vi "Smoothing.vi"(9 "Data in":T1) -> (1 "Data out":T1)   [LabVIEW 2013]
uses:
  xcontrol/Interface VIs/Interface typedefs/Interface-Data array.ctl
  xcontrol/Interface VIs/Interface typedefs/Interface-Data format definition.ctl
  xcontrol/Typedefs/Xctl-XY data type definition.ctl
  xcontrol/Typedefs/Xctrl-ROI type enum.ctl
  <vilib>/Analysis/3filter.llb/IIR Filter with I.C. (DBL).vi
  Global variables/gl_Functional Imaging-Global variables.vi
  <vilib>/Analysis/NI_AALBase.lvlib
  xcontrol/XGrapher.xctl
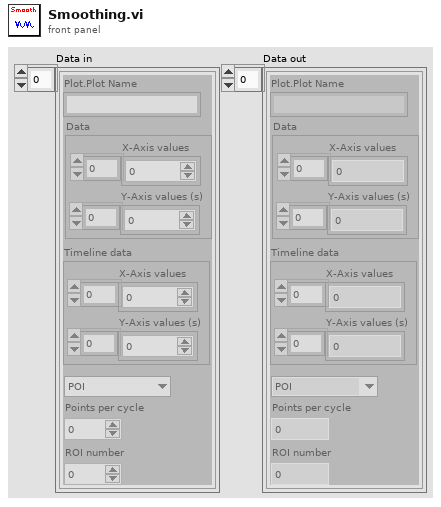
[diagram p1: front panel]
types:
  T1 = typedef "Interface-Data array.ctl" = T2[]
  T2 = typedef "Interface-Data format definition.ctl" = cluster{"Plot.Plot Name":string, "Data":T3, "Timeline data":T3, "Type":T4, "Points per cycle":u16, "ROI number":u16}
  T3 = typedef "XGrapher.xctl/Xctl-XY data type definition.ctl" = cluster{"X-Axis values":sgl[], "Y-Axis values (s)":i32[]}
  T4 = typedef "Xctrl-ROI type enum.ctl" = enum16{"POI", "Mini-scan", "Group"}
  T5 = typedef "Functional Imging UI Refs.ctl" = cluster{"Menu ref":refnum<k9>, "Image control":refnum<vi>, "VI ref":refnum<vi>, "XGrapher":refnum<vi>, "Smoothing":refnum<vi>, "POI Averaging":refnum<vi>, "Normalize":refnum<vi>, "POI data points in each trial":refnum<vi>, "Channel":refnum<vi>, "Experiment data folder path":refnum<vi>, "[ROI vis]":refnum<vi>, "[Groups] visbl":T6, "Group Name":refnum<vi>, "POI index":refnum<vi>, "Trial No.":refnum<vi>, "Intensity Zoom":refnum<vi>, "Trial Cursor Enabled":refnum<vi>, "Number of Trials (ind 1)":refnum<vi>, "Number of Trials (ind 2)":refnum<vi>, "MiniScans Available":refnum<vi>, "POI Available":refnum<vi>, "Defer graph updates":refnum<vi>, "Waveform selector":refnum<vi>, "#of selected POI":refnum<vi>, "#of selected MiniScans":refnum<vi>, "#of selected groups":refnum<vi>, "Max Z-Projection":refnum<vi>, "Z-Plane Selector":refnum<vi>, "Index of miniscan point to visualise":refnum<vi>, "ROI vis. mode":refnum<vi>, "Total # of points":refnum<vi>, "Index of group clicked on":refnum<vi>, "Pane 1":refnum<vi>, "Pane 2":refnum<vi>, "Pane 3":refnum<vi>, "Pane 4":refnum<vi>, "Pane 5":refnum<vi>, "Pane 6":refnum<vi>, "Deselect all ROI":refnum<vi>, "Deselect all groups":refnum<vi>}
  T6 = typedef "Groups array referecne.ctl" = refnum<vi>
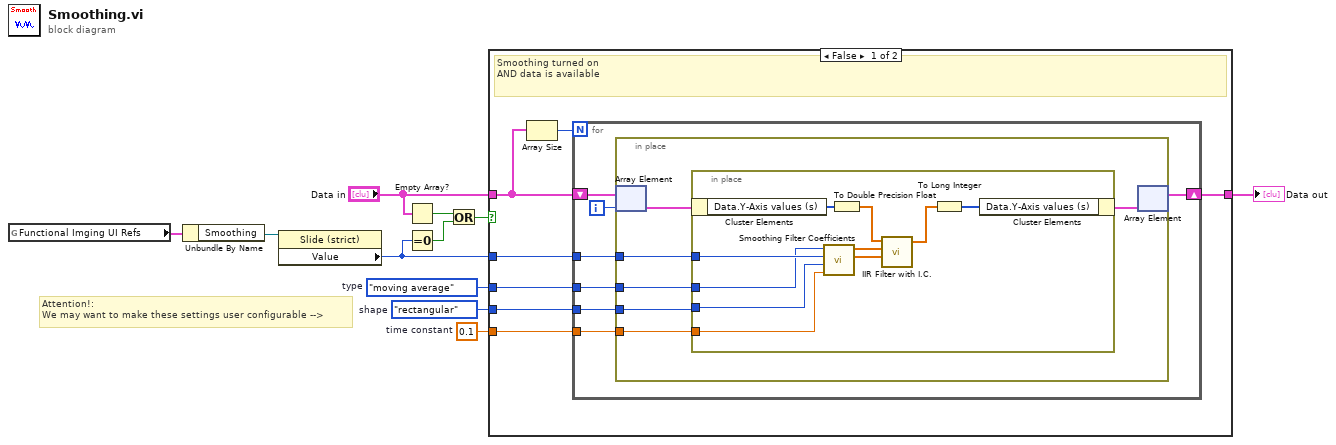
[diagram p0: block diagram]
diagram:
  w2 = 0.1  # time constant
  w3 = enum16{"rectangular", "triangular"}."rectangular"  # shape
  w4 = enum16{"moving average", "exponential"}."moving average"  # type
  # "Attention!:\nWe may want to make these settings user configurable -->"
  n1 = global read "gl_Functional Imaging-Global variables.vi" "Functional Imging UI Refs"() -> (w1:T5)
  n2 = Unbundle By Name(w1) -> ("Smoothing"=w11:refnum<vi>)
  n3 = property on="Property Node" class="Slide (strict)"(reference=w11) -> ("Value"=w5:i32)  [unwired: 1 in, 2 out]
  n4 = Empty Array?(array="Data in") -> (empty?=w8:bool)
  n5 = Equal To 0?(x=w5) -> (x = 0?=w9:bool)
  n6 = Or(x=w8, y=w9) -> (x .or. y?=w10:bool)
  n7 = case shown="False" w10 {
    tunnel: w5 -> [w18 _]
    tunnel: "Data in" -> [w12 w42]
    tunnel: [w17 w42] -> w6
    tunnel: w4 -> [w16 _]
    tunnel: w3 -> [w15 _]
    tunnel: w2 -> [w14 _]
    frame False {
      # "Smoothing turned on\nAND data is available"
      n8 = Array Size(array=w12) -> (size(s)=w13:i32)
      n9 = for {
        N: w13 -> [_]
        tunnel: w18 -> [w25]
        tunnel: w16 -> [w24]
        tunnel: w15 -> [w23]
        tunnel: w14 -> [w22]
        shift-right: [w20] -> w17
        shift-left: w12 -> [w19]
        i -> [w21]
        n10 = in-place {
          in-place-border: w25 -> [w31]
          in-place-border: w24 -> [w30]
          in-place-border: w23 -> [w29]
          in-place-border: w22 -> [w28]
          n11 = in-place-array #1(w19, w21) -> (w27:T2)
          n12 = in-place {
            in-place-border: w31 -> [w39]
            in-place-border: w30 -> [w36]
            in-place-border: w29 -> [w35]
            in-place-border: w28 -> [w34]
            n13 = in-place-cluster #2(w27) -> ("Data.Y-Axis values (s)"=w38:i32[])
            n14 = call <vilib>:"Smoothing Filter Coefficients.vi"("time constant"=w34, "shape"=w35, "half-width"=w39, "type"=w36) -> ("forward coefficients"=w41:dbl[], "reverse coefficients"=w40:dbl[])  [unwired: 5 in, 1 out]
            n15 = To Double Precision Float(number=w38) -> (double precision float=w33:dbl[])
            n16 = call-poly <vilib>:"IIR Filter with I.C..vi"("Forward Coefficients"=w41, "Reverse Coefficients"=w40, "X"=w33) -> ("Filtered X"=w37:dbl[])  [unwired: 4 in, 3 out]
            n17 = To Long Integer(number=w37) -> (32bit integer=w32:i32[])
            n18 = in-place-cluster #2("Data.Y-Axis values (s)"=w32) -> (w26:T2)
          }
          n19 = in-place-array #1(w26) -> (w20:T1)  [unwired: 1 out]
        }
      }
    }
    frame True {
      # "Smoothing set to zero\nOR no data available"
    }
  }
  "Data out" <- w6
